vi "Test_Create.vi"(0 "reference in":refnum<class "Test.lvclass">, 2 "Engine":bool, 3 "Dyno":bool, 5 "error in (no error)":errorcluster) -> (14 "reference out":refnum<class "Test.lvclass">, 19 "error out":errorcluster)   [LabVIEW 2024, in "Test.lvclass"]
uses:
  Test.lvclass
  Test.lvclass/Test.ctl
panel:
  # "Connector Pane"
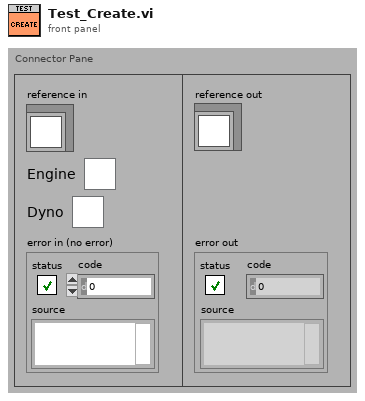
[diagram p1: front panel]
types:
  T1 = typedef "Test.lvclass/ObjectAttributes.ctl" = cluster{"Engine":bool, "Dynamometer":bool, "Test Status":enum16{"Test Start", "Test Continue", "Test Failed", "Test Success"}, "History String":string}
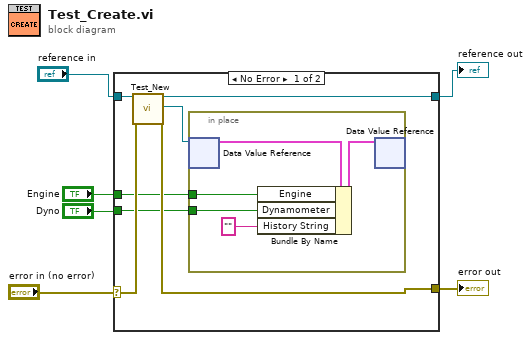
[diagram p0: block diagram]
diagram:
  n1 = case shown="No Error" "error in (no error)" {
    selector: "error in (no error)" -> [w12 w20]
    tunnel: [w10 w20] -> w5
    tunnel: "reference in" -> [w13 w19]
    tunnel: [w11 w19] -> w3
    tunnel: "Engine" -> [w8 _]
    tunnel: "Dyno" -> [w7 _]
    frame No Error {
      n2 = call "Test_New.vi"("reference in"=w13, "error in (no error)"=w12) -> ("reference out"=w11:refnum<class "Test.lvclass">, "DVRRefOut"=w9:refnum<data-value>, "error out"=w10:errorcluster)  [unwired: 14 in, 1 out]
      n3 = in-place {
        in-place-border: w8 -> [w16]
        in-place-border: w7 -> [w15]
        n4 = in-place-dvr #1(w9) -> (w18:T1)  [unwired: 1 out]
        n5 = Bundle By Name(cluster=w18, "Engine"=w16, "Dynamometer"=w15, "History String"="") -> (w17:T1)
        n6 = in-place-dvr #1(w17) -> ()  [unwired: 2 out]
      }
    }
    frame Error {
    }
  }
  "error out" <- w5
  "reference out" <- w3
